vi "List Roles.vi"(8 "error in (no error)":errorcluster, 11 "IAM Session in":refnum<class "IAM Session.lvclass">) -> (0 "error out":errorcluster, 2 "Roles":T1[](array[typedef]), 3 "IAM Session out":refnum<class "IAM Session.lvclass">)   [LabVIEW 2015, in "NI_AWS_IAM.lvlib" / "IAM Session.lvclass"]
uses:
  IAM Session.lvclass
  Role.ctl
  Core/HTTP Request/Request Options.ctl
  Core/HTTP Request/Name Value Pair.ctl
  Core/HTTP Request/Region handling.ctl
  Core/HTTP Request/URL formatting.ctl
  Core/HTTP Request/HTTP Request.lvclass
  XML Parsing/NI_XML Parsing.lvlib
  NI_AWS_IAM.lvlib
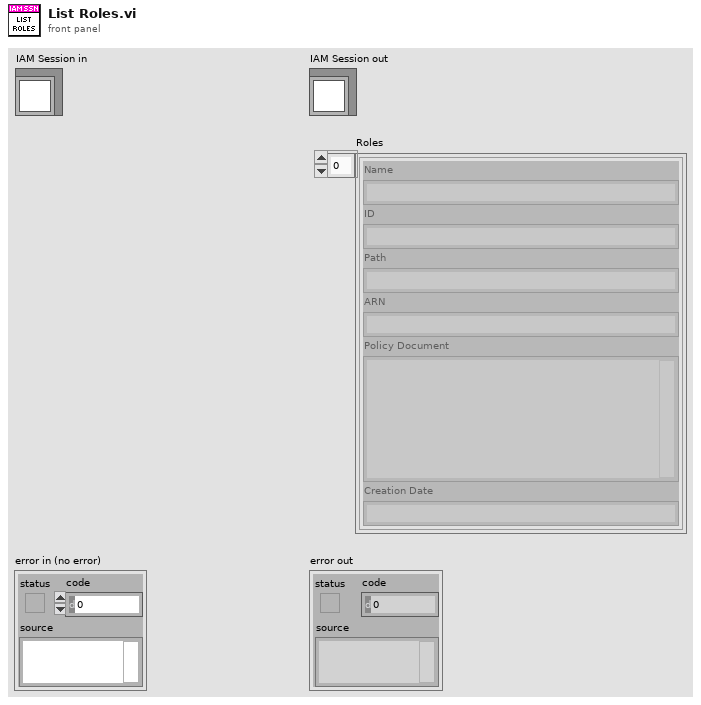
[diagram p1: front panel]
types:
  T1 = typedef "NI_AWS_IAM.lvlib/Role.ctl" = cluster{"Name":string, "ID":string, "Path":string, "ARN":string, "Policy Document":string, "Creation Date":string}
  T2 = typedef "NI_AWS_Core.lvlib/HTTP Request.lvclass/Name Value Pair.ctl" = cluster{"name":string, "value":string}
  T3 = typedef "NI_AWS_Core.lvlib/HTTP Request.lvclass/Request Options.ctl" = cluster{"request headers":T2[], "request parameters":T2[], "request body":string, "region handling":T4, "URL formatting":T5}
  T4 = typedef "NI_AWS_Core.lvlib/HTTP Request.lvclass/Region handling.ctl" = enum16{"use region everywhere", "use region (authentication only)", "use region (URL only)", "ignore region everwhere"}
  T5 = typedef "NI_AWS_Core.lvlib/HTTP Request.lvclass/URL formatting.ctl" = enum16{"region-", "region."}
  T6 = typedef "NI_AWS_Core.lvlib/HTTP Request.lvclass/Response.ctl" = cluster{"Headers":string, "Body":string}
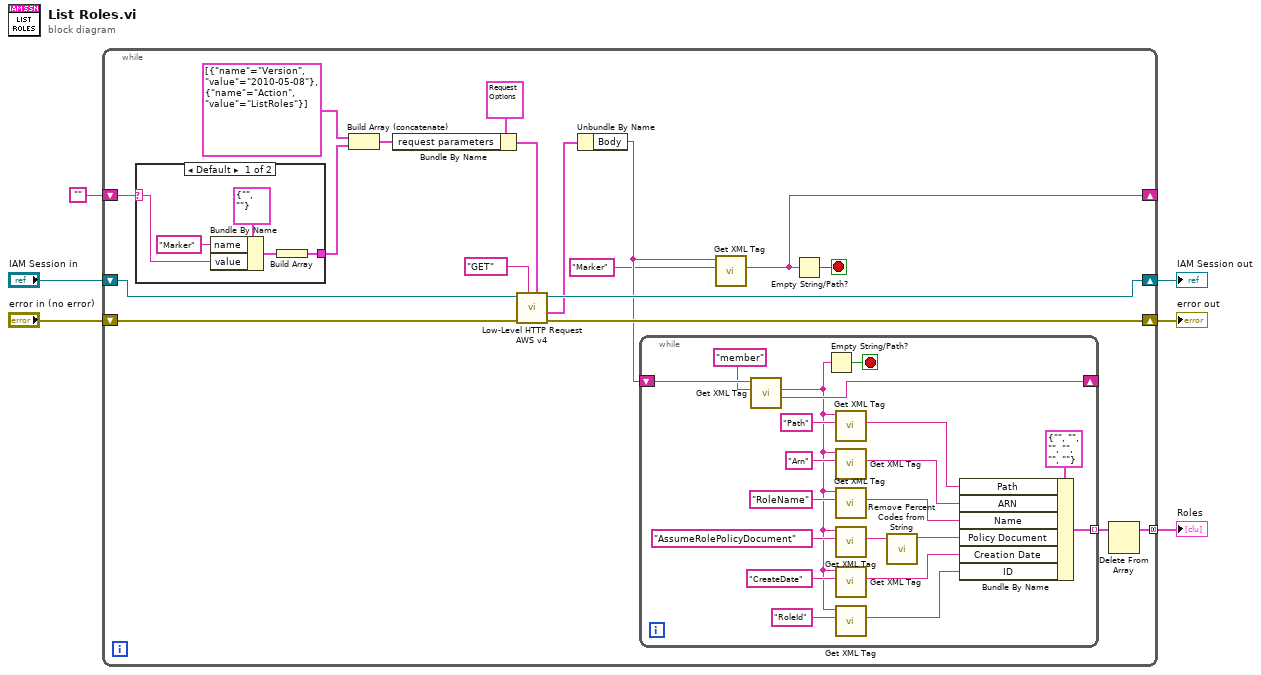
[diagram p0: block diagram]
diagram:
  n1 = while {
    shift-right: [w23] -> w5
    shift-left: "error in (no error)" -> [w24]
    shift-right: [w22] -> w4
    shift-left: "IAM Session in" -> [w21]
    shift-right: [w11] -> _
    shift-left: "" -> [w15]
    tunnel: [w8] -> w1 mode=concatenating
    stop <- w10 stop-if-true
    n2 = case shown="Default" w15 {
      selector: w15 -> [w27 _]
      tunnel: [w25 _] -> w14
      frame Default {
        n3 = Bundle By Name(cluster=T2 {"name"="", "value"=""} ("Name Value Pair"), "name"="Marker", "value"=w27) -> (w26:T2)
        n4 = Build Array(w26) -> (w25:T2[])
      }
      frame "" {
      }
    }
    n5 = Build Array (concatenate)(T2[] [{"name"="Version", "value"="2010-05-08"}, {"name"="Action", "value"="ListRoles"}], w14) -> (w18:T2[])
    n6 = Bundle By Name(cluster=T3 {"request headers"=[], "request parameters"=[], "request body"="", "region handling"=enum."use region everywhere", "URL formatting"=enum."region."} ("Request Options"), "request parameters"=w18) -> (w19:T3)
    n7 = call "Low-Level HTTP Request AWS v4.vi"("Request Options"=w19, "HTTP-Verb"="GET", "error in (no error)"=w24, "AWS Core in"=w21) -> ("error out"=w23:errorcluster, "Response"=w16:T6, "AWS Core out"=w22:refnum<class "IAM Session.lvclass">)  [unwired: 4 in, 1 out]
    n8 = Unbundle By Name(w16) -> ("Body"=w13:string)
    n9 = while {
      shift-right: [w47] -> _
      shift-left: w13 -> [w49]
      tunnel: [w45] -> w9 mode=indexing
      stop <- w46 stop-if-true
      n10 = call "Get XML Tag.vi"("Tag name"="member", "XML String in"=w49) -> ("Remaining string"=w47:string, "Tag value"=w34:string)  [unwired: 5 in, 3 out]
      n11 = Empty String/Path?(string/path=w34) -> (empty?=w46:bool)
      n12 = call "Get XML Tag.vi"("Tag name"="Path", "XML String in"=w34) -> ("Tag value"=w38:string)  [unwired: 5 in, 4 out]
      n13 = call "Get XML Tag.vi"("Tag name"="Arn", "XML String in"=w34) -> ("Tag value"=w37:string)  [unwired: 5 in, 4 out]
      n14 = call "Get XML Tag.vi"("Tag name"="RoleName", "XML String in"=w34) -> ("Tag value"=w36:string)  [unwired: 5 in, 4 out]
      n15 = call "Get XML Tag.vi"("Tag name"="AssumeRolePolicyDocument", "XML String in"=w34) -> ("Tag value"=w31:string)  [unwired: 5 in, 4 out]
      n16 = call "Get XML Tag.vi"("Tag name"="CreateDate", "XML String in"=w34) -> ("Tag value"=w35:string)  [unwired: 5 in, 4 out]
      n17 = call "Get XML Tag.vi"("Tag name"="RoleId", "XML String in"=w34) -> ("Tag value"=w32:string)  [unwired: 5 in, 4 out]
      n18 = call "Remove Percent Codes from String.vi"("String in"=w31) -> ("String out"=w30:string)  [unwired: 10 in]
      n19 = Bundle By Name(cluster=T1 {"Name"="", "ID"="", "Path"="", "ARN"="", "Policy Document"="", "Creation Date"=""} ("Role"), "Path"=w38, "ARN"=w37, "Name"=w36, "Policy Document"=w30, "Creation Date"=w35, "ID"=w32) -> (w45:T1)
    }
    n20 = call "Get XML Tag.vi"("Tag name"="Marker", "XML String in"=w13) -> ("Tag value"=w11:string)  [unwired: 5 in, 4 out]
    n21 = Empty String/Path?(string/path=w11) -> (empty?=w10:bool)
    n22 = Delete From Array(array=w9) -> (array with subset deleted=w8:T1[])  [unwired: 2 in, 1 out]
  }
  "error out" <- w5
  "IAM Session out" <- w4
  "Roles" <- w1
